vi "SysDef.Rename.vi"(7 "Force Rename (F)":bool, 8 "error in (no error)":errorcluster, 10 "Name":string, 11 "nodeID":u64) -> (0 "error out":errorcluster, 2 "Success?":bool, 3 "nodeID out":u64)   [LabVIEW 2016, in "Advanced System Definition.lvlib"]
uses:
  Advanced System Definition.lvlib
  NationalInstruments.VeriStand.SystemDefinitionAPI
  <vilib>/NI VeriStand/Custom Device API/Custom Device API.lvlib
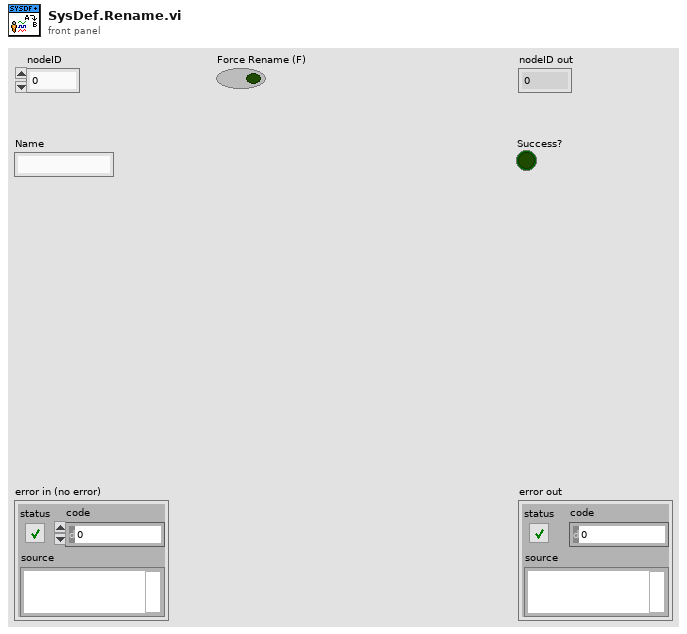
[diagram p1: front panel]
types:
  T1 = typedef "Custom Device API.lvlib/Custom Device Item Ref.ctl" = u64
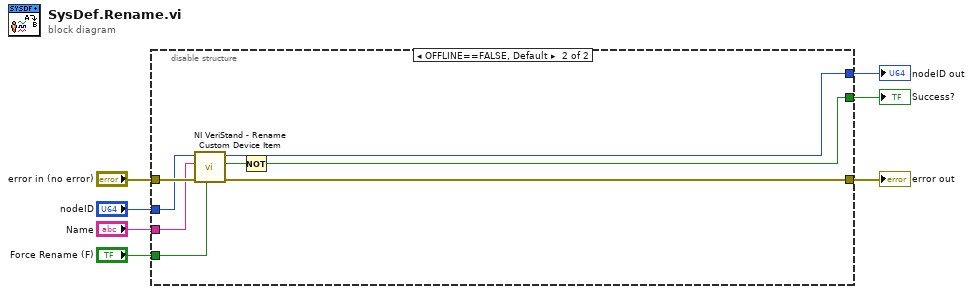
[diagram p0: block diagram]
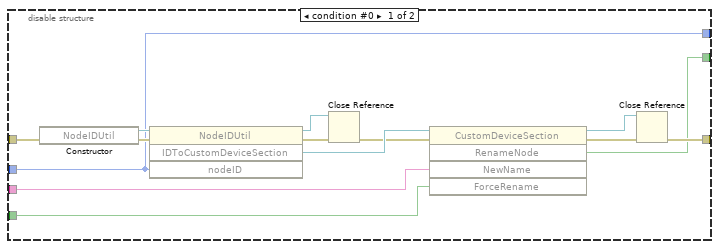
[diagram p2: hidden frame]
diagram:
  n1 = disable-structure shown="OFFLINE==FALSE, Default" {
    disable-tunnel: "nodeID" -> [w11 w28]
    disable-tunnel: "error in (no error)" -> [w18 w29]
    disable-tunnel: [w10 w25] -> w6
    disable-tunnel: "Name" -> [w12 w27]
    disable-tunnel: [w9 w23] -> w4
    disable-tunnel: [w11 w24] -> w2
    disable-tunnel: "Force Rename (F)" -> [w8 w22]
    frame condition #0 {
      n2 = constructor class="NodeIDUtil"(error in=w18) -> (reference out=w20:refnum<k24>, error out=w19:errorcluster)  [unwired: 2 in, 1 out]
      n3 = invoke class="NodeIDUtil" method="IDToCustomDeviceSection"(reference=w20, error in=w19, "nodeID"=w11) -> (reference out=w17:refnum<k24>, error out=w14:errorcluster, "IDToCustomDeviceSection"=w21:refnum<k24>)  [unwired: 1 in, 1 out]
      n4 = Close Reference(reference=w17, error in (no error)=w14) -> (error out=w13:errorcluster)
      n5 = invoke class="CustomDeviceSection" method="RenameNode"(reference=w21, error in=w13, "NewName"=w12, "ForceRename"=w8) -> (reference out=w15:refnum<k24>, error out=w16:errorcluster, "RenameNode"=w9:bool)  [unwired: 1 in, 2 out]
      n6 = Close Reference(reference=w15, error in (no error)=w16) -> (error out=w10:errorcluster)
    }
    frame condition #1 (active) {
      n7 = call <vilib>:"NI VeriStand - Rename Custom Device Item.vi"("Force Rename (F)"=w22, "error in (no error)"=w29, "New Name"=w27, "Item Ref in"=w28) -> ("error out"=w25:errorcluster, "Request invalid?"=w26:bool, "Item Ref out"=w24:T1)  [unwired: 5 in]
      n8 = Not(x=w26) -> (.not. x?=w23:bool)
    }
  }
  "nodeID out" <- w2
  "error out" <- w6
  "Success?" <- w4
